vi "Epilogue.vi"() -> ()   [LabVIEW 2016]
panel:
  in  "Stop Button":bool
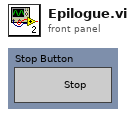
[diagram p1: front panel]
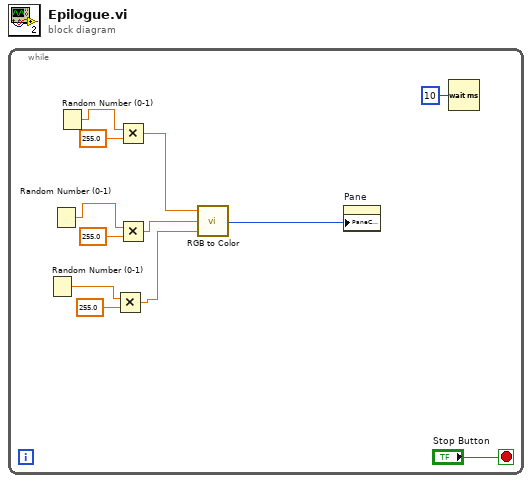
[diagram p0: block diagram]
diagram:
  n1 = while {
    stop <- "Stop Button" stop-if-true
    n2 = Random Number (0-1)() -> (number: 0 to 1=w9:dbl)
    n3 = Random Number (0-1)() -> (number: 0 to 1=w7:dbl)
    n4 = Random Number (0-1)() -> (number: 0 to 1=w8:dbl)
    n5 = Multiply(x=w9, y=255.0) -> (x*y=w3:dbl)
    n6 = Multiply(x=w8, y=255.0) -> (x*y=w5:dbl)
    n7 = Multiply(x=w7, y=255.0) -> (x*y=w4:dbl)
    n8 = call <vilib>:"RGB to Color.vi"("B"=w3, "G"=w4, "R"=w5) -> ("Color"=w2:u32)
    n9 = property on="Pane" class="Pane"("PaneColor"=w2) -> ()  [unwired: 2 in, 2 out]
    n10 = Wait (ms)(milliseconds to wait=u32 10) -> ()  [unwired: 1 out]
  }
